vi "MissionRecieveTest.vi"() -> ()   [LabVIEW 2013]
uses:
  Data/TypeDefs/MissionTypeControl.ctl
  Data/TypeDefs/UTM Location.ctl
  RIO-OCU_Comm/ToRIO.ctl
  Classes/Missions/GenericMission/GenericMission.lvclass
  RIO-OCU_Comm/NetworkStreams/Reader/NetworkStreamReader.lvclass
panel:
  out "Connected?":bool
  out "error out":errorcluster
  out "Points of Interest":T1[](array[typedef]) {"North" format="%#_10f"; "East" format="%#_8f"}
  out "Mission Type":T2
  in  "stop":bool
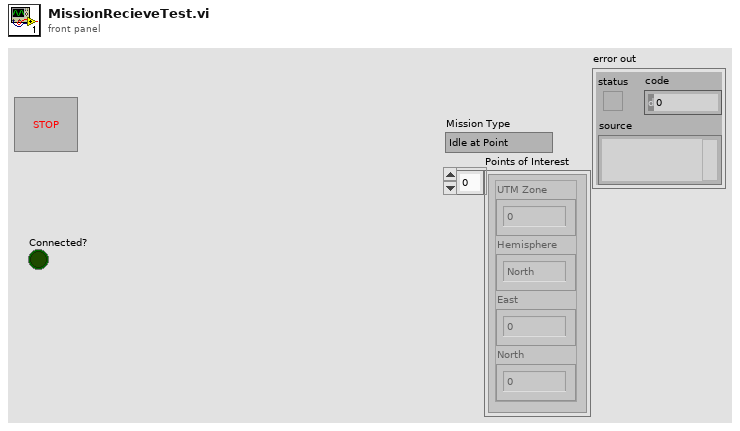
[diagram p1: front panel]
types:
  T1 = typedef "UTM Location.ctl" = cluster{"UTM Zone":dbl, "Hemisphere":enum16{"North", "South"}, "East":dbl, "North":dbl}
  T2 = typedef "MissionTypeControl.ctl" = enum16{"Idle at Point", "Drive to Waypoint", "Round Buoy to Port", "Round Buoy to Starboard", "Pass Between Buoys", "Station Keeping"}
  T3 = typedef "ToRIO.ctl" = cluster{"Mission":refnum<class "GenericMission.lvclass">}
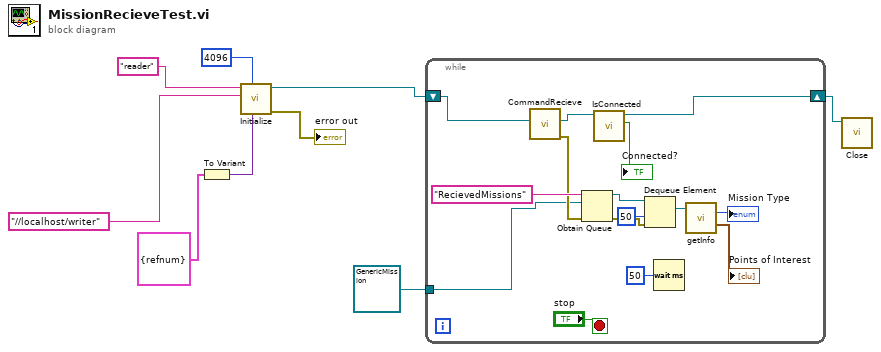
[diagram p0: block diagram]
diagram:
  n1 = To Variant(anything=T3 {"Mission"=refnum} ("To RIO")) -> (Variant=w8:variant)
  n2 = call "Initialize.vi"("Default return"=w8, "reader buffer size"=4096, "writer url"="//localhost/writer", "reader name"="reader" ("format string")) -> ("error out"=→"error out":errorcluster, "NetworkStreamWriter out"=w7:refnum<class "NetworkStreamReader.lvclass">)  [unwired: 6 in]
  n3 = while {
    shift-right: [w10] -> w5
    shift-left: w7 -> [w12]
    tunnel: refnum<class "GenericMission.lvclass"> refnum ("Mission") -> [w18]
    stop <- "stop" stop-if-true
    n4 = call "CommandRecieve.vi"("NetworkStreamReader in"=w12) -> ("error out"=w22:errorcluster, "NetworkStreamReader out"=w11:refnum<class "NetworkStreamReader.lvclass">)  [unwired: 9 in]
    n5 = Obtain Queue(name (unnamed)="RecievedMissions", element data type=w18, error in (no error)=w22) -> (queue out=w21:refnum<queue>, error out=w20:errorcluster)  [unwired: 2 in, 1 out]
    n6 = call "IsConnected.vi"("NetworkStreamReader in"=w11) -> ("Connected?"=→"Connected?":bool, "NetworkStreamReader out"=w10:refnum<class "NetworkStreamReader.lvclass">)  [unwired: 8 in, 1 out]
    n7 = Dequeue Element(queue=w21, timeout in ms (-1)=50, error in (no error)=w20) -> (element=w16:refnum<class "GenericMission.lvclass">)  [unwired: 3 out]
    n8 = Wait (ms)(milliseconds to wait=u32 50) -> ()  [unwired: 1 out]
    n9 = call-dynamic "getInfo.vi"("GenericMission in"=w16) -> ("Mission Type"=→"Mission Type":T2, "Points of Interest"=→"Points of Interest":T1[])  [unwired: 6 in, 7 out]
  }
  n10 = call "Close.vi"("NetworkStreamReader in"=w5) -> ()  [unwired: 10 in, 1 out]
